vi "RunStatistics.vi"() -> ()   [LabVIEW 2018]
uses:
  General Libraries/statistics/StatisticsControl.ctl
  <vilib>/Utility/miscctls.llb/LVPointDoubleTypeDef.ctl
  General Libraries/statistics/OutputSelection.ctl
  typedef/StateMachineControl.ctl
  typedef/AcquisitionFrame.ctl
  Read and Save Files/FileType.ctl
  VisionLibrariesXimea/xiLib/xiLIB_64bit/xiLIB/xiCamLib/xiCam/PRM/PRM/PRM_v2.ctl
  VisionLibrariesXimea/xiLib/xiLIB_64bit/xiLIB/xiCamLib/xiCam/PRM/ACQ_TIMING_MODE/ACQ_TIMING_MODE.ctl
  C:/XIMEA/API/x64/xiApi.NETX64.dll
  General Libraries/statistics.lvlib
  General Libraries/Photon Filtering.lvlib
  General Libraries/myFFT.lvlib
  Read and Save Files/RW_Protocols.lvlib
panel:
  out "r":dbl[][][](array[numeric])
  out "ready for stat ?":bool
  in  "N average":i32=10
  out "error out":errorcluster
  in  "output type":T1
  in  "phase multiple select":i32[](listbox)=[0, 1, 2, 3]
  in  "Tab Control":T2(tab)
  in  "subimage control":T4={"2^n : x"=10, "2^n : y"=10, "lower left box Position"={"X"=1752.0, "Y"=1167.0}, "Height"=100, "Width"=100} {"2^n : y" min=1 max=13; "2^n : x" min=1 max=13}
  out "time for acquire":dbl[unit]
  out "Intensity Graph 2":u16[][](graph)
  out "FFT":dbl[][](graph)
  out "filtered  FFT":dbl[][](graph)
  in  "save stats":bool
  in  "image stat":T5
  out "Intensity Graph":dbl[][](graph)
  out "total frames":i32
  in  "Hologram array":dbl[](array[numeric])=[0.0, 0.25, 0.5, 0.75]
  out "fft cluster":T6
  in  "Run statistics":bool
  in  "Stop Button":bool
  # "edit this array to define how the hologram is implmented. For example, H = I1 - I3 + i I2 - i I3 will be define by the default value"
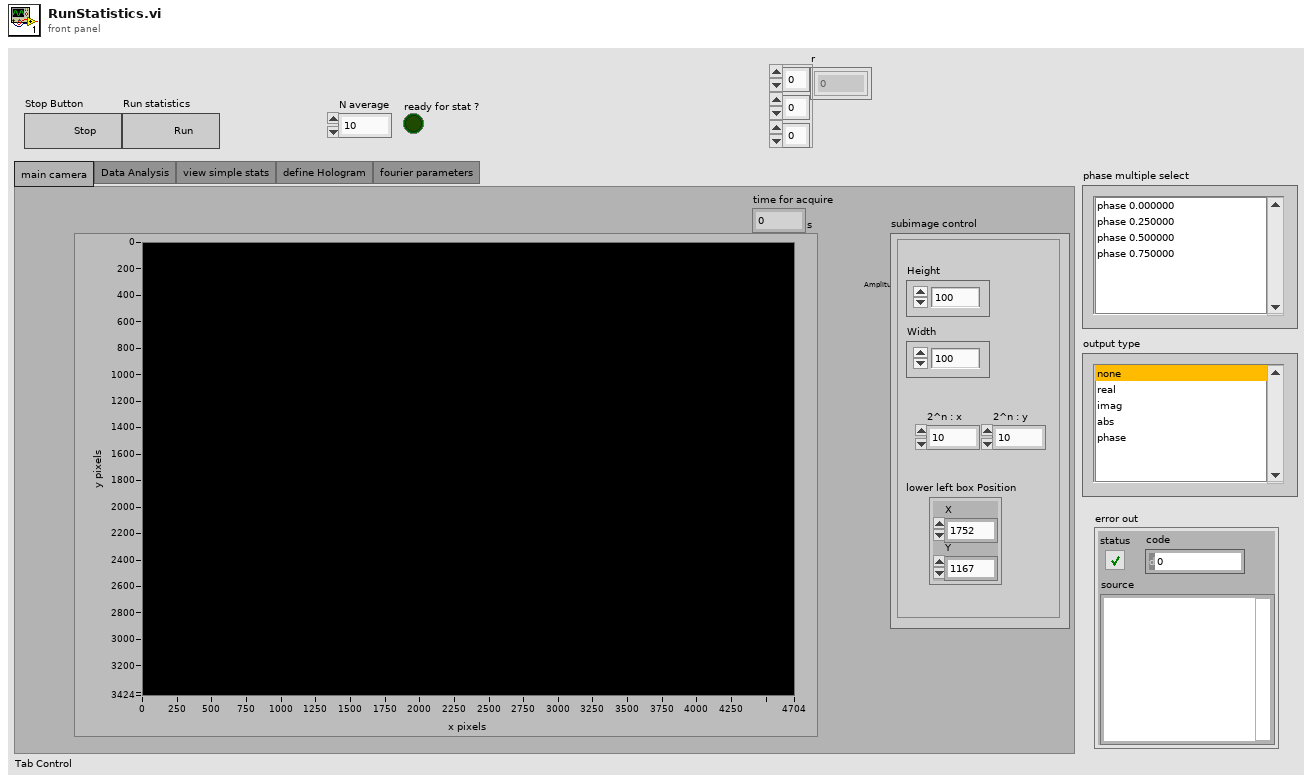
[diagram p1: front panel]
types:
  T1 = typedef "statistics.lvlib/OutputSelection.ctl" = i32
  T2 = enum32{"main camera", "Data Analysis", "view simple stats", "define Hologram", "fourier parameters"}
  T3 = typedef "LVPointDoubleTypeDef.ctl" = cluster{"X":dbl, "Y":dbl}
  T4 = cluster{"2^n : x":i8, "2^n : y":i8, "lower left box Position":T3, "Height":i32, "Width":i32}
  T5 = typedef "statistics.lvlib/StatisticsControl.ctl" = enum16{"var", "image", "SNR", "std", "average"}
  T6 = cluster{"dFx":dbl, "dFy":dbl, "Nx":i32, "Ny":i32, "FxMax":dbl, "FyMax":dbl, "Xwidth":dbl, "Ywidth":dbl, "dx":dbl, "dy":dbl, "Fx points":dbl[], "X points":dbl[], "Y points":dbl[], "Fy points":dbl[]}
  T7 = typedef "AcquisitionFrame.ctl" = cluster{"data array":u8[], "nframe":i32, "sframe":i32, "nframe0":i32, "data format":i32, "is sequence running ?":bool, "timestamp":dbl}
  T8 = typedef "StateMachineControl.ctl" = enum16{"stop acquire", "acquire sequence", "wait", "start acquire sequence", "start acquire", "acquire"}
  T9 = typedef "PRM_v2.ctl" = enum16{"ACQ_BUFFER_SIZE", "ACQ_FRAME_BURST_COUNT", "ACQ_TIMING_MODE", "ACQ_TRANSPORT_BUFFER_SIZE", "AE_MAX_LIMIT", "AEAG", "AEAG_LEVEL", "API_VERSION", "AG_MAX_LIMIT", "APPLY_CMS", "AUTO_BANDWIDTH_CALCULATION", "AUTO_WB", "AVAILABLE_BANDWIDTH", "AVAILABLE_BANDWIDTH_MAX", "AVAILABLE_BANDWIDTH_MIN", "BPC", "BUFFER_POLICY", "BUFFERS_QUEUE_SIZE", "CC_MATRIX_00", "CC_MATRIX_01", "CC_MATRIX_02", "CC_MATRIX_03", "CC_MATRIX_10", "CC_MATRIX_11", "CC_MATRIX_12", "CC_MATRIX_13", "CC_MATRIX_20", "CC_MATRIX_21", "CC_MATRIX_22", "CC_MATRIX_23", "CC_MATRIX_30", "CC_MATRIX_31", "CC_MATRIX_32", "CC_MATRIX_33", "CHIP_TEMP", "CMS", "COLOR_FILTER_ARRAY", "COOLING", "DEBOUNCE_EN", "DEBOUNCE_POL", "DEBOUNCE_T0", "DEBOUNCE_T1", "DEBUG_LEVEL", "DEFAULT_CC_MATRIX", "DEVICE_INSTANCE_PATH", "DEVICE_MODEL_ID", "DEVICE_NAME", "DEVICE_SN", "DEVICE_TYPE", "DEVICE_USER_ID", "DOWNSAMPLING", "DOWNSAMPLING_MAX", "DOWNSAMPLING_MIN", "DOWNSAMPLING_TYPE", "DRV_VERSION", "EXP_PRIORITY", "EXPOSURE", "EXPOSURE_DIRECT_UPDATE", "EXPOSURE_MAX", "EXPOSURE_MIN", "FFS_FILE_NAME", "FPGA1_VERSION", "FRAMERATE", "FRAMERATE_MAX", "FRAMERATE_MIN", "FREE_FFS_SIZE", "GAIN", "GAIN_DIRECT_UPDATE", "GAIN_MAX", "GAIN_MIN", "GAMMAC", "GAMMAY", "GPI_LEVEL", "GPI_MODE", "GPI_SELECTOR", "GPI_SELECTOR_MAX", "GPI_SELECTOR_MIN", "GPO_MODE", "GPO_SELECTOR", "GPO_SELECTOR_MAX", "GPO_SELECTOR_MIN", "HDR", "HDR_T1", "HDR_T2", "HEIGHT", "HEIGHT_MAX", "HEIGHT_MIN", "HOUSE_TEMP", "IMAGE_DATA_FORMAT", "IMAGE_IS_COLOR", "INPUT_CMS_PROFILE", "IS_COOLED", "IS_DEVICE_EXIST", "KNEEPOINT1", "KNEEPOINT2", "LED_MODE", "LED_SELECTOR", "LED_SELECTOR_MAX", "LED_SELECTOR_MIN", "LIMIT_BANDWIDTH", "LIMIT_BANDWIDTH_MAX", "LIMIT_BANDWIDTH_MIN", "LUT_EN", "LUT_INDEX", "LUT_INDEX_MAX", "LUT_INDEX_MIN", "LUT_VALUE", "LUT_VALUE_MAX", "LUT_VALUE_MIN", "MANUAL_WB", "MCU1_VERSION", "MCU2_VERSION", "OFFSET_X", "OFFSET_X_MAX", "OFFSET_X_MIN", "OFFSET_Y", "OFFSET_Y_MAX", "OFFSET_Y_MIN", "OUTPUT_CMS_PROFILE", "OUTPUT_DATA_BIT_DEPTH", "OUTPUT_DATA_PACKING", "READ_FILE_FFS", "RECENT_FRAME", "SENSOR_DATA_BIT_DEPTH", "SENSOR_MODE", "SENSOR_TAPS", "SHARPNESS", "SHUTTER_TYPE", "TARGET_TEMP", "TRG_DELAY", "TRG_SELECTOR", "TRG_SOFTWARE", "TRG_SOURCE", "USED_FFS_SIZE", "WB_KB", "WB_KG", "WB_KR", "WIDTH", "WIDTH_MAX", "WIDTH_MIN", "WRITE_FILE_FFS", "ACQ_BUFFER_SIZE_UNIT", "ACQ_TRANSPORT_BUFFER_COMMIT", "AEAG_ROI_HEIGHT", "AEAG_ROI_OFFSET_X", "AEAG_ROU_OFFSET_Y", "AEAG_ROI_WIDTH", "API_CONTEXT_LIST", "BINNING_HORIZONTAL", "BINNING_SELECTOR", "BINNING_VERTICAL", "COLUMN_FPN_CORRECTION", "COUNTER_SELECTOR", "COUNTER_VALUE", "DECIMATION_HORIZONTAL", "DECIMATION_SELECTOR", "DECIMATION_VERTICAL", "DEVICE_ID", "DEVICE_LOCATION_PATH", "DEVICE_MANIFEST", "DEVICE_RESET", "DEVICE_SENS_SN", "EXPOSURE_BURST_COUNT", "FFS_ACCESS_KEY", "GAIN_SELECTOR", "HW_REVISION", "IMAGE_BLACK_LEVEL", "IMAGE_DATA_BIT_DEPTH", "IMAGE_DATA_FORMAT_RGB32_ALPHA", "IMAGE_PAYLOAD_SIZE", "LENS_APERTURE_VALUE", "LENS_FEATURE", "LENS_FEATURE_SELECTOR", "LENS_FOCAL_LENGTH", "LENS_FOCUS_DISTANCE", "LENS_FOCUS_MOVE", "LENS_FOCUS_MOVEMENT_VALUE", "LENS_MODE", "OUTPUT_DATA_PACKING_TYPE", "SENSOR_CLOCK_FREQ_HZ", "SENSOR_CLOCK_FREQ_INDEX", "SENSOR_FEATURE_SELECTOR", "SENSOR_FEATURE_VALUE", "SENSOR_OUTPUT_CHANNEL_COUNT", "TRANSPORT_PIXEL_FORMAT", "TS_RST_MODE", "TS_RST_SOURCE"}
  T10 = typedef "ACQ_TIMING_MODE.ctl" = enum16{"FREE_RUN", "FRAME_RATE"}
  T11 = typedef "RW_Protocols.lvlib/FileType.ctl" = enum16{"png", "csv", "tiff", "dat", "bin", "txt"}
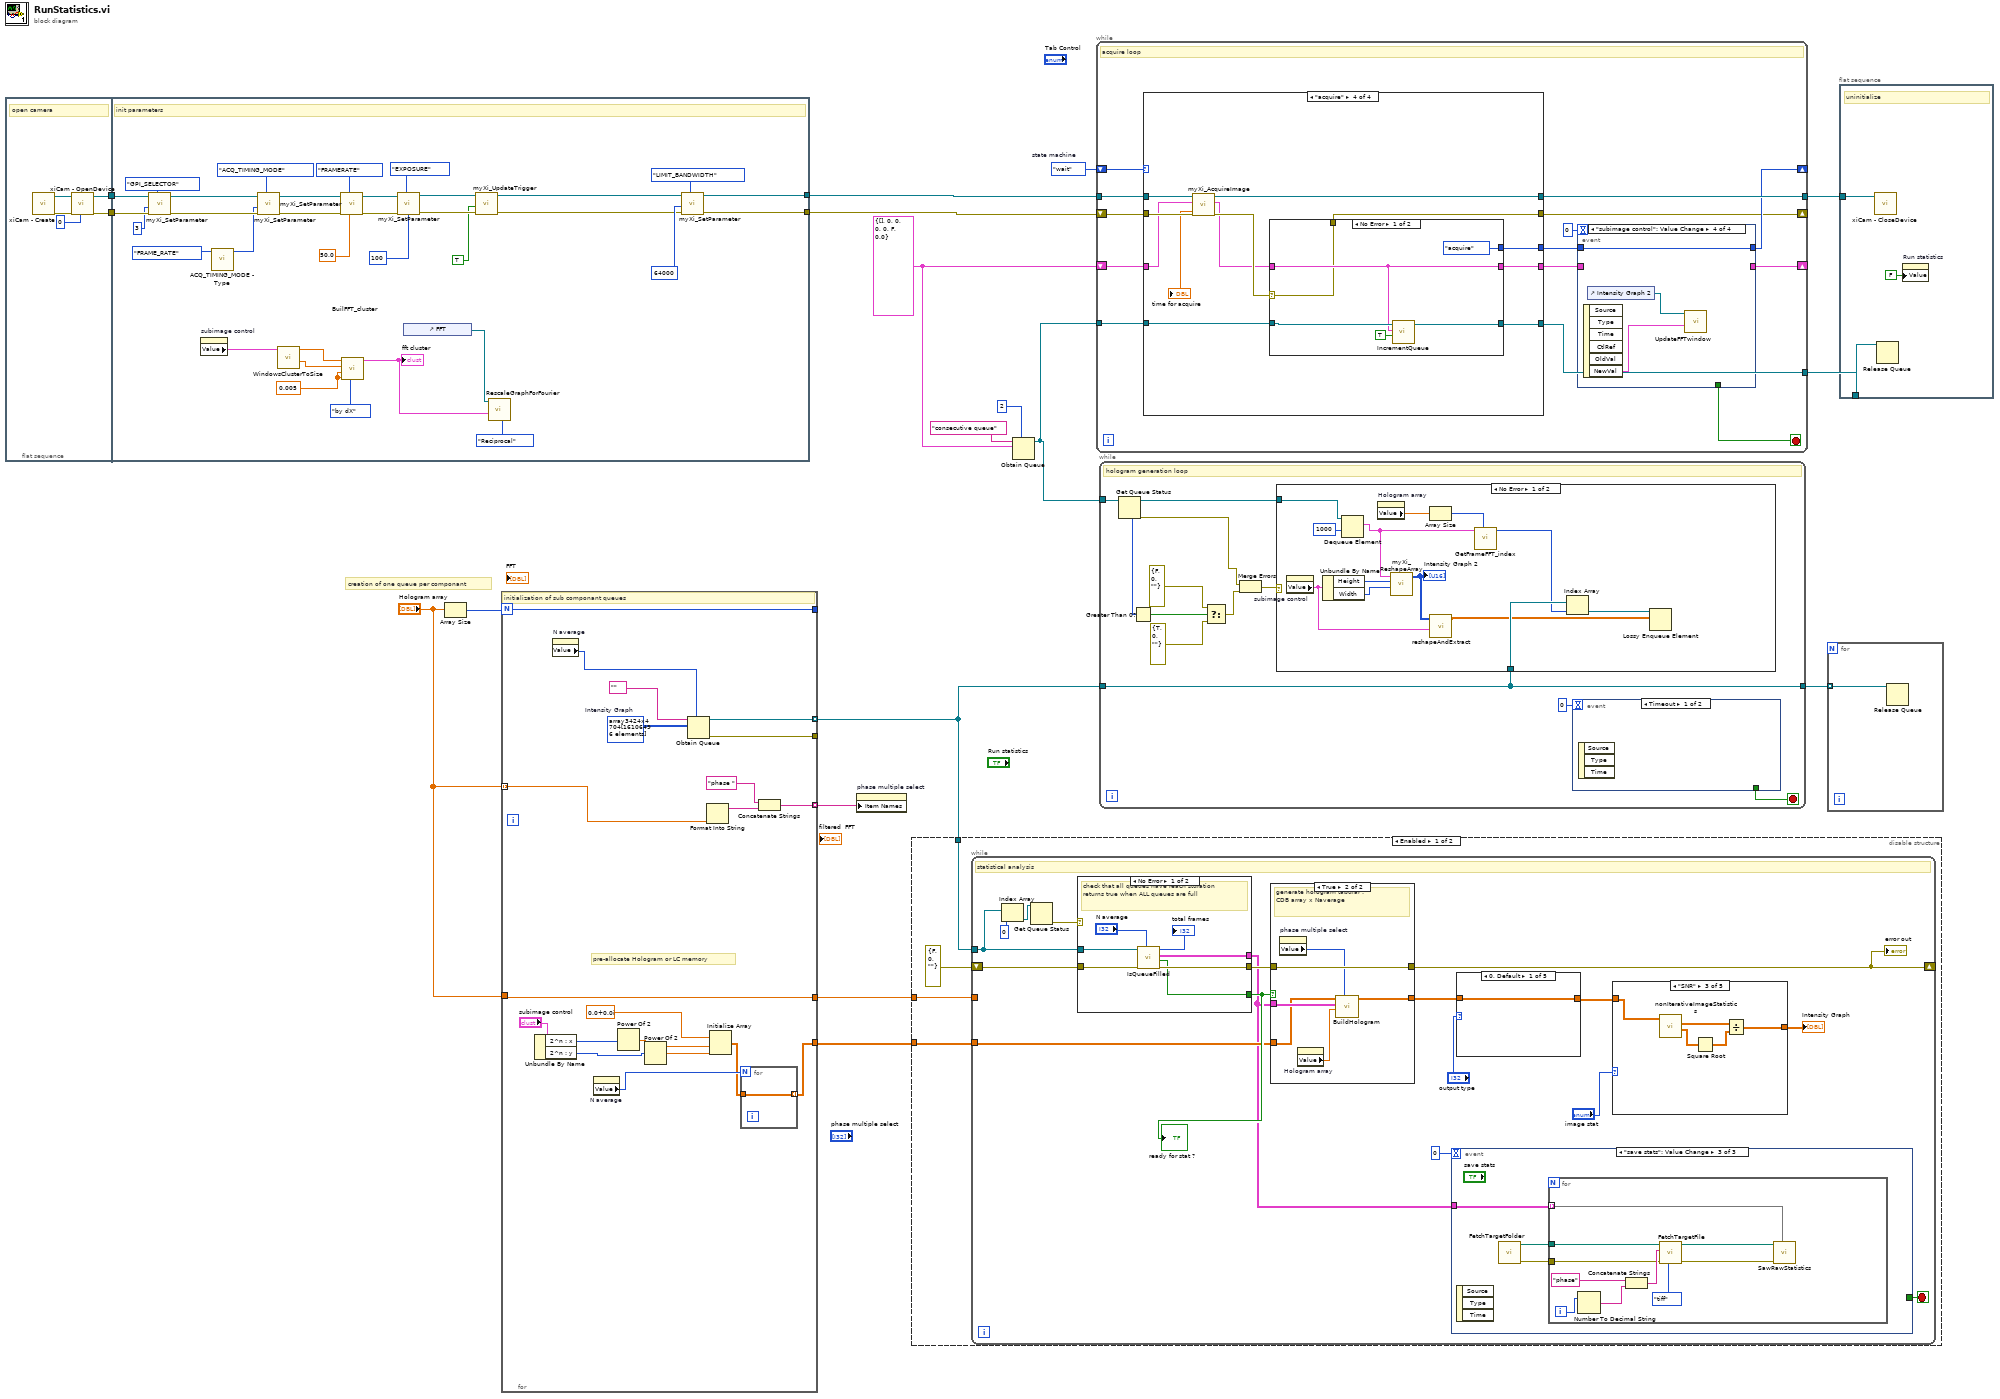
[diagram p0: block diagram]
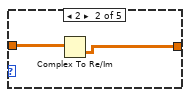
[diagram p2: hidden frame]
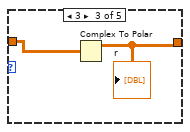
[diagram p3: hidden frame]
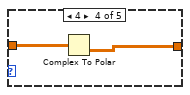
[diagram p4: hidden frame]
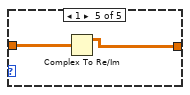
[diagram p5: hidden frame]
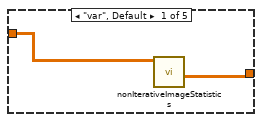
[diagram p6: hidden frame]
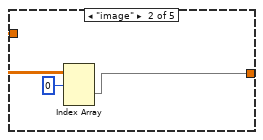
[diagram p7: hidden frame]
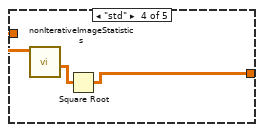
[diagram p8: hidden frame]
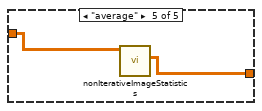
[diagram p9: hidden frame]
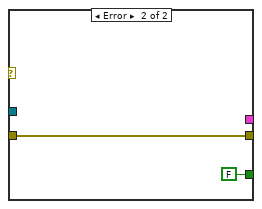
[diagram p11: hidden frame]
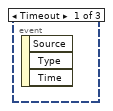
[diagram p12: hidden frame]
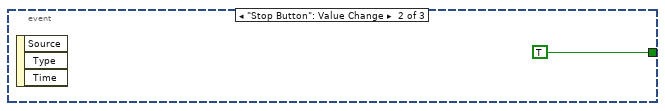
[diagram p13: hidden frame]
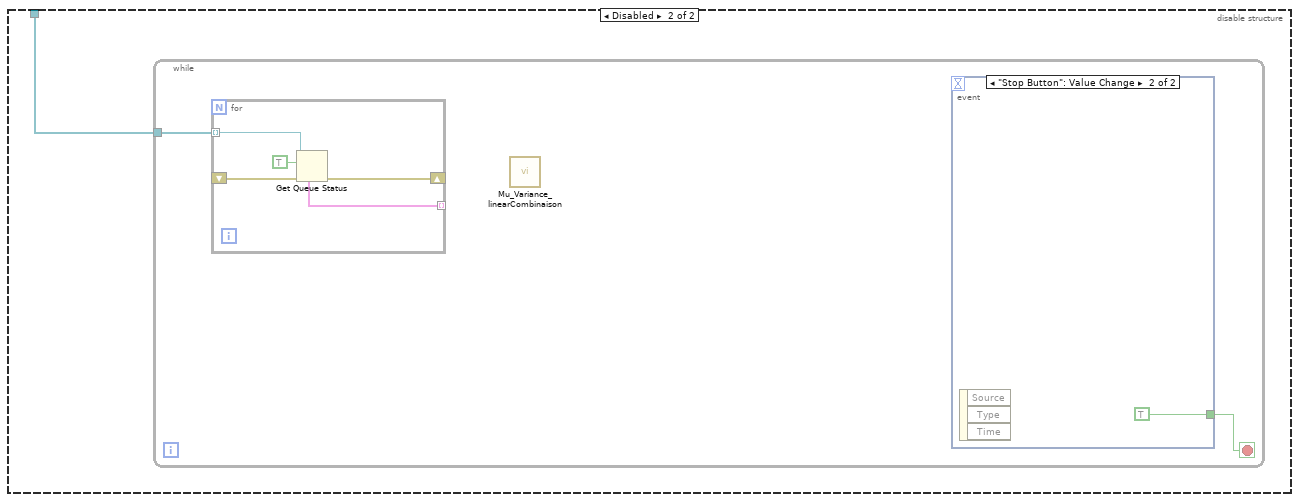
[diagram p14: hidden frame]
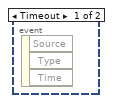
[diagram p15: hidden frame]
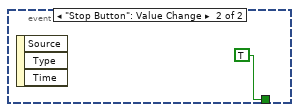
[diagram p17: hidden frame]
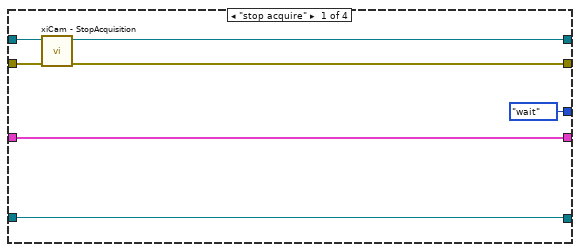
[diagram p18: hidden frame]
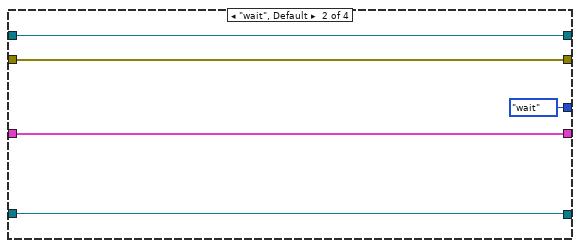
[diagram p19: hidden frame]
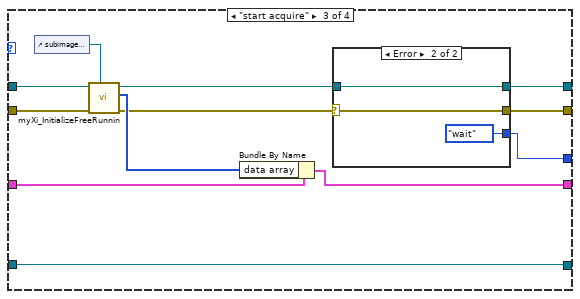
[diagram p20: hidden frame]
diagram:
  w1 = T7 {"data array"=[], "nframe"=0, "sframe"=0, "nframe0"=0, "data format"=0, "is sequence running ?"=FALSE, "timestamp"=0.0} ("acquisition frame")
  w13 = StateMachineControl."wait"  # state machine
  # "creation of one queue per componant"
  n1 = flat-sequence {
    tunnel: [w20] -> w18
    tunnel: [w19] -> w17
    tunnel: w18 -> [w56]
    tunnel: w17 -> [w57]
    tunnel: [w33] -> w16
    tunnel: [w34] -> w15
    frame #0 {
      # "open camera"
      n2 = call "xiCam - Create.vi"() -> ("error out"=w22:errorcluster, "new xiCam"=w23:refnum<k24>)  [unwired: 10 in]
      n3 = call "xiCam - OpenDevice.vi"("DevID"=0, "error in (no error)"=w22, "xiCam In"=w23) -> ("error out"=w19:errorcluster, "xiCam Out"=w20:refnum<k24>)  [unwired: 7 in]
    }
    frame #1 {
      w31 = 0.005 ("input X")
      # "init parameters"
      n4 = call "myXi_SetParameter.vi"("input PRM"=PRM_v2."GPI_SELECTOR", "error in"=w57, "input value I32"=i64 3, "xiCam IN"=w56) -> ("error out"=w53:errorcluster, "xiCam Out"=w52:refnum<k24>)  [unwired: 6 in]
      n5 = property on="subimage control" class="Clust (strict)"() -> ("Value"=w25:T4)  [unwired: 2 in, 2 out]
      n6 = call "ACQ_TIMING_MODE - Type.vi"("ACQ TIMING MODE"=ACQ_TIMING_MODE."FRAME_RATE") -> ("ACQ_TIMING_MODE_VALUE"=w50:i32)  [unwired: 9 in, 1 out]
      n7 = call "myXi_SetParameter.vi"("input PRM"=PRM_v2."ACQ_TIMING_MODE", "error in"=w53, "input value I32"=w50, "xiCam IN"=w52) -> ("error out"=w43:errorcluster, "xiCam Out"=w44:refnum<k24>)  [unwired: 6 in]
      n8 = call "WindowsClusterToSize.vi"("subwindow control 2"=w25) -> ("Ny"=w30:dbl, "Nx"=w29:dbl)  [unwired: 9 in]
      n9 = call "myXi_SetParameter.vi"("input value DBL"=sgl 50.0, "input PRM"=PRM_v2."FRAMERATE", "error in"=w43, "xiCam IN"=w44) -> ("error out"=w41:errorcluster, "xiCam Out"=w42:refnum<k24>)  [unwired: 6 in]
      n10 = call "BuilFFT_cluster.vi"("Enum"=enum16{"by dF", "by dX"}."by dX", "input Y"=w31, "input X"=w31, "Ny"=w30, "Nx"=w29) -> ("fft cluster"=w27:T6)  [unwired: 6 in]
      "fft cluster" <- w27
      n11 = call "myXi_SetParameter.vi"("input PRM"=PRM_v2."EXPOSURE", "error in"=w41, "input value I32"=i64 100, "xiCam IN"=w42) -> ("error out"=w39:errorcluster, "xiCam Out"=w40:refnum<k24>)  [unwired: 6 in]
      n12 = control-ref of="FFT"() -> (w24:refnum<vi>)
      n13 = call "myXi_UpdateTrigger.vi"("error in (no error)"=w39, "trigger"=TRUE, "xiCam IN"=w40) -> ("error out"=w35:errorcluster, "xiCam Out"=w32:refnum<k24>)  [unwired: 7 in]
      n14 = call "RescaleGraphForFourier.vi"("fft reference"=w24, "fft cluster"=w27, "Enum"=enum16{"Reciprocal", "Real"}."Reciprocal") -> ()  [unwired: 8 in]
      n15 = call "myXi_SetParameter.vi"("input PRM"=PRM_v2."LIMIT_BANDWIDTH", "error in"=w35, "input value I32"=i64 64000, "xiCam IN"=w32) -> ("error out"=w34:errorcluster, "xiCam Out"=w33:refnum<k24>)  [unwired: 6 in]
    }
  }
  n16 = Array Size(array="Hologram array") -> (size(s)=w8:i32)
  n17 = for {
    N: w8 -> [w70]
    tunnel: [w77] -> w6 mode=indexing
    tunnel: [w75] -> _
    tunnel: [w73] -> w5 mode=indexing
    tunnel: [w70] -> _
    tunnel: "Hologram array" -> [w69]
    tunnel: [w69] -> w4
    tunnel: "Hologram array" -> [w68] mode=indexing
    tunnel: [w63] -> w2
    w74 = u16[][] array3424x4704[16106496 elements]  # Intensity Graph
    # "pre-allocate Hologram or LC memory"
    # "initialization of sub componant queues"
    n18 = Unbundle By Name("subimage control") -> ("2^n : x"=w62:i8, "2^n : y"=w60:i8)
    n19 = property on="N average" class="DigNum (strict)"() -> ("Value"=w58:i32)  [unwired: 2 in, 2 out]
    n20 = property on="N average" class="DigNum (strict)"() -> ("Value"=w65:i32)  [unwired: 2 in, 2 out]
    n21 = Power Of 2(x=w62) -> (2^x=w61:dbl)
    n22 = Power Of 2(x=w60) -> (2^x=w59:dbl)
    n23 = Obtain Queue(max queue size (-1, unlimited)=w58, name (unnamed)="", element data type=w74) -> (queue out=w77:refnum<queue>, error out=w75:errorcluster)  [unwired: 2 in, 1 out]
    n24 = Format Into String(w68) -> (resulting string=w72:string)  [unwired: 3 in, 1 out]
    n25 = Initialize Array(cdb 0.0+0.0i, w61, w59) -> (w64:cdb[][])
    n26 = for {
      N: w65 -> [_]
      tunnel: w64 -> [w78]
      tunnel: [w78] -> w63 mode=indexing
    }
    n27 = Concatenate Strings("phase ", w72) -> (w73:string)
  }
  n28 = property on="phase multiple select" class="LstBox (strict)"("Item Names"=w5) -> ()  [unwired: 2 in, 2 out]
  n29 = disable-structure shown="Enabled" {
    disable-tunnel: w6 -> [w82 w155]
    disable-tunnel: w4 -> [w81 _]
    disable-tunnel: w2 -> [w79 _]
    frame Enabled {
      n30 = while {
        tunnel: w82 -> [w96]
        shift-right: [w90] -> _
        shift-left: errorcluster {"status"=FALSE, "code"=0, "source"=""} ("error out") -> [w97]
        tunnel: w81 -> [_]
        tunnel: w79 -> [w89]
        stop <- w98 stop-if-true
        # "statistical analysis"
        n31 = Index Array(array=w96, index=0) -> (element=w94:refnum<queue>)
        n32 = Get Queue Status(queue=w94) -> (error out=w93:errorcluster)  [unwired: 2 in, 7 out]
        n33 = case shown="No Error" w93 {
          tunnel: w97 -> [w138 w140]
          tunnel: [w137 w140] -> w91
          tunnel: w96 -> [w132 _]
          tunnel: [w135 FALSE ("ready for stat ?")] -> w92
          tunnel: [w134 _] -> w83
          frame No Error {
            # "check that all queues have reach sturation\nreturns true when ALL queues are full"
            n34 = call "IsQueueFilled.vi"("N average"="N average", "error in (no error)"=w138, "Array 2"=w132) -> ("error out"=w137:errorcluster, "ready for stat ?"=w135:bool, "elements"=w134:cluster{"Intensity Graph 3":u8[][]}[][], "sum"=→"total frames":i32)  [unwired: 5 in]
          }
          frame Error {
          }
        }
        "ready for stat ?" <- w92
        n35 = case shown="True" w92 {
          tunnel: w91 -> [w125 w131]
          tunnel: [w125 w131] -> w90
          tunnel: w89 -> [w124 w127]
          tunnel: [w124 w129] -> w84
          tunnel: w83 -> [_ w128]
          frame False {
          }
          frame True {
            # "generate hologram tabular :\nCDB array x Naverage"
            n36 = property on="phase multiple select" class="LstBox (strict)"() -> ("Value"=w130:i32[])  [unwired: 2 in, 2 out]
            n37 = property on="Hologram array" class="Arr (strict)"() -> ("Value"=w126:dbl[])  [unwired: 2 in, 2 out]
            n38 = call "BuildHologram.vi"("phase multiple select"=w130, "Hologram array"=w126, "elements"=w128, "pre-allocated HOL"=w127) -> ("HOL out"=w129:cdb[][][])  [unwired: 7 in]
          }
        }
        "error out" <- w90
        n39 = event shown="[2] \"save stats\": Value Change" {
          selector: _ -> [_ _ _]
          dyn-events: _ -> [_ _ _]
          timeout: 0 -> [_ _ _]
          tunnel: [_ TRUE _] -> w98
          tunnel: w83 -> [_ _ w144]
          event Timeout {
            n40 = event-data() -> ()  [unwired: 1 in, 3 out]
          }
          event "Stop Button": Value Change {
            n41 = event-data() -> ()  [unwired: 1 in, 3 out]
          }
          event "save stats": Value Change {
            n42 = event-data() -> ()  [unwired: 1 in, 3 out]
            n43 = call "FetchTargetFolder.vi"() -> ("error out"=w142:errorcluster, "Full File Path"=w143:path)  [unwired: 10 in]
            n44 = for {
              tunnel: w144 -> [w146] mode=indexing
              tunnel: w143 -> [w149]
              tunnel: w142 -> [w150]
              i -> [w154]
              n45 = Number To Decimal String(number=w154) -> (decimal integer string=w152:string)  [unwired: 1 in]
              n46 = Concatenate Strings("phase", w152) -> (w151:string)
              n47 = call "FetchTargetFile.vi"("file type"=FileType."tiff", "error in (no error)"=w150, "FileName"=w151, "Target Folder"=w149) -> ("error out"=w147:errorcluster, "Full File Path"=w148:path)  [unwired: 6 in]
              n48 = call "SawRawStatistics.vi"("elements 2"=w146, "error in (no error)"=w147, "Full File Path"=w148) -> ()  [unwired: 8 in, 1 out]
            }
          }
        }
        n49 = case shown="0, Default" "output type" {
          tunnel: w84 -> [w100 w102 w104 w106 w107]
          tunnel: [w100 w101 w103 w105 w108] -> w85
          frame 0, Default {
          }
          frame 2 {
            n50 = Complex To Re/Im(x + iy=w102) -> (y=w101:dbl[][][])  [unwired: 1 out]
          }
          frame 3 {
            n51 = Complex To Polar(r * e^(i*theta)=w104) -> (r=w103:dbl[][][])  [unwired: 1 out]
            "r" <- w103
          }
          frame 4 {
            n52 = Complex To Polar(r * e^(i*theta)=w106) -> (theta=w105:dbl[][][])  [unwired: 1 out]
          }
          frame 1 {
            n53 = Complex To Re/Im(x + iy=w107) -> (x=w108:dbl[][][])  [unwired: 1 out]
          }
        }
        n54 = case shown="\"SNR\"" "image stat" {
          tunnel: [w109 w111 w114 w119 w122] -> w87
          tunnel: w85 -> [w110 w113 w118 w121 w123]
          frame "var", Default {
            n55 = call "nonIterativeImageStatistics.vi"("HOL in"=w110) -> ("var n+1"=w109:dbl[][])  [unwired: 9 in, 1 out]
          }
          frame "image" {
            n56 = Index Array(array=w113, index (dim 0)=0 ("index (page)")) -> (element=w111:cdb[][])  [unwired: 2 in]
          }
          frame "SNR" {
            n57 = call "nonIterativeImageStatistics.vi"("HOL in"=w118) -> ("var n+1"=w117:dbl[][], "MU n+1"=w116:dbl[][])  [unwired: 9 in]
            n58 = Square Root(x=w117) -> (sqrt(x)=w115:dbl[][])
            n59 = Divide(x=w116, y=w115) -> (x/y=w114:dbl[][])
          }
          frame "std" {
            n60 = call "nonIterativeImageStatistics.vi"("HOL in"=w121) -> ("var n+1"=w120:dbl[][])  [unwired: 9 in, 1 out]
            n61 = Square Root(x=w120) -> (sqrt(x)=w119:dbl[][])
          }
          frame "average" {
            n62 = call "nonIterativeImageStatistics.vi"("HOL in"=w123) -> ("MU n+1"=w122:dbl[][])  [unwired: 9 in, 1 out]
          }
        }
        "Intensity Graph" <- w87
      }
    }
    frame Disabled {
      n63 = while {
        tunnel: w155 -> [w156]
        stop <- w157 stop-if-true
        n64 = for {
          tunnel: w156 -> [w162] mode=indexing
          shift-right: [w159] -> _
          shift-left: _ -> [w160]
          tunnel: [w158] -> _ mode=indexing
          n65 = Get Queue Status(queue=w162, return elements? (F)=TRUE, error in (no error)=w160) -> (error out=w159:errorcluster, elements=w158:cluster{"Intensity Graph":u16[][]}[])  [unwired: 6 out]
        }
        n66 = call "Mu_Variance_linearCombinaison.vi"() -> ()  [unwired: 12 in]
        n67 = event shown="[1] \"Stop Button\": Value Change" {
          selector: _ -> [_ _]
          dyn-events: _ -> [_ _]
          timeout: _ -> [_ _]
          tunnel: [_ TRUE] -> w157
          event Timeout {
            n68 = event-data() -> ()  [unwired: 1 in, 3 out]
          }
          event "Stop Button": Value Change {
            n69 = event-data() -> ()  [unwired: 1 in, 3 out]
          }
        }
      }
    }
  }
  n70 = Obtain Queue(max queue size (-1, unlimited)=2, name (unnamed)="consecutive queue", element data type=w1) -> (queue out=w10:refnum<queue>)  [unwired: 2 in, 2 out]
  n71 = while {
    tunnel: w16 -> [w173]
    tunnel: [w172] -> w14
    shift-right: [w167] -> _
    shift-left: w13 -> [w175]
    shift-right: [w170] -> _
    shift-left: w1 -> [w171]
    shift-right: [w164] -> _
    shift-left: w15 -> [w174]
    tunnel: w10 -> [w166]
    tunnel: [w165] -> w11
    stop <- w177 stop-if-true
    # "acquire loop"
    n72 = case shown="\"acquire\"" w175 {
      tunnel: w174 -> [w182 w187 w201 w220]
      tunnel: w173 -> [w183 w186 w199 w221]
      tunnel: [w181 w186 w198 w219] -> w172
      tunnel: w171 -> [w184 w189 w197 w218]
      tunnel: [w184 w189 w196 w214] -> w169
      tunnel: [StateMachineControl."wait" ("state machine") StateMachineControl."wait" ("state machine") w195 w216] -> w168
      tunnel: [w180 w187 w194 w210] -> w164
      tunnel: w166 -> [w178 w185 w193 w213]
      tunnel: [w178 w185 w193 w212] -> w165
      frame "stop acquire" {
        n73 = call "xiCam - StopAcquisition.vi"("error in (no error)"=w182, "xiCam In"=w183) -> ("error out"=w180:errorcluster, "xiCam Out"=w181:refnum<k24>)  [unwired: 8 in]
      }
      frame "wait", Default {
      }
      frame "start acquire" {
        n74 = control-ref of="subimage control"() -> (w192:refnum<vi>)
        n75 = call "myXi_InitializeFreeRunnin.vi"("subimage IN"=w192, "error in (no error)"=w201, "xiCam IN"=w199) -> ("error out"=w190:errorcluster, "Array"=w191:u8[], "xiCam Out"=w200:refnum<k24>)  [unwired: 6 in]
        n76 = Bundle By Name(cluster=w197, "data array"=w191) -> (w196:T7)
        n77 = case shown="Error" w190 {
          selector: w190 -> [w203 w208]
          tunnel: w200 -> [w206 w209]
          tunnel: [w205 w209] -> w198
          tunnel: [w204 StateMachineControl."wait" ("state machine")] -> w195
          tunnel: [w202 w208] -> w194
          frame No Error {
            w204 = StateMachineControl."acquire"  # state machine
            n78 = invoke class="xiCam" method="StartAcquisition"(reference=w206, error in=w203) -> (reference out=w205:refnum<k24>, error out=w202:errorcluster)  [unwired: 1 in, 1 out]
          }
          frame Error {
          }
        }
      }
      frame "acquire" {
        n79 = call "myXi_AcquireImage.vi"("error in"=w220, "acquisition frame"=w218, "xiCam In"=w221) -> ("error out"=w217:errorcluster, "acquisition frame out"=w215:T7, "xiCam Out"=w219:refnum<k24>, "time for acquire"=→"time for acquire":dbl[unit])  [unwired: 4 in, 1 out]
        n80 = case shown="No Error" w217 {
          selector: w217 -> [w222 w229]
          tunnel: [StateMachineControl."acquire" ("state machine") w230] -> w216
          tunnel: w215 -> [w224 w233]
          tunnel: [w224 w233] -> w214
          tunnel: w213 -> [w226 w232]
          tunnel: [w223 w232] -> w212
          tunnel: [w222 w228] -> w210
          frame No Error {
            n81 = call "IncrementQueue.vi"("is sequence running ?"=TRUE, "acquisition frame"=w224, "queue in"=w226) -> ("queue out"=w223:refnum<queue>)  [unwired: 8 in]
          }
          frame Error {
            n82 = Unbundle By Name(w229) -> ("code"=w231:i32)
            n83 = case shown="1172" w231 {
              tunnel: [StateMachineControl."wait" ("state machine") StateMachineControl."acquire" ("state machine")] -> w230
              tunnel: w229 -> [w234 _]
              tunnel: [w234 errorcluster {"status"=FALSE, "code"=0, "source"=""} ("error IO")] -> w228
              frame 0, Default {
              }
              frame 1172 {
              }
            }
          }
        }
      }
    }
    n84 = event shown="[3] \"subimage control\": Value Change" {
      selector: _ -> [_ _ _ _]
      dyn-events: _ -> [_ _ _ _]
      timeout: 0 -> [_ _ _ _]
      tunnel: [_ TRUE _ _] -> w177
      tunnel: [w238 w240 w244 _] -> w170
      tunnel: w169 -> [w238 w240 w244 _]
      tunnel: w168 -> [w239 _ _ w250]
      tunnel: [w239 StateMachineControl."wait" ("state machine") w243 w250] -> w167
      event Timeout {
        n85 = event-data() -> ()  [unwired: 1 in, 3 out]
      }
      event "Stop Button": Value Change {
        n86 = event-data() -> ()  [unwired: 1 in, 6 out]
      }
      event "Run statistics": Value Change {
        n87 = event-data() -> ("NewVal"=w245:bool)  [unwired: 1 in, 5 out]
        n88 = case shown="True" w245 {
          tunnel: [w246 StateMachineControl."start acquire" ("state machine")] -> w243
          frame False {
            w246 = StateMachineControl."stop acquire"  # state machine
          }
          frame True {
          }
        }
      }
      event "subimage control": Value Change {
        n89 = event-data() -> ("NewVal"=w249:T4)  [unwired: 1 in, 5 out]
        n90 = control-ref of="Intensity Graph 2"() -> (w248:refnum<vi>)
        n91 = call "UpdateFFTwindow.vi"("subwindow IN"=w249, "Intensity Graph"=w248) -> ()  [unwired: 9 in, 1 out]
      }
    }
  }
  n92 = while {
    tunnel: w10 -> [w257]
    tunnel: w6 -> [w253]
    tunnel: [w253] -> w7
    stop <- w261 stop-if-true
    # "hologram generation loop"
    n93 = Get Queue Status(queue=w257) -> (queue out=w254:refnum<queue>, error out=w252:errorcluster, # elements in queue=w255:i32)  [unwired: 2 in, 5 out]
    n94 = Greater Than 0?(x=w255) -> (x > 0?=w260:bool)
    n95 = Select(t=errorcluster {"status"=FALSE, "code"=0, "source"=""} ("error constant"), s=w260, f=errorcluster {"status"=TRUE, "code"=0, "source"=""} ("error constant")) -> (s? t:f=w251:errorcluster)
    n96 = Merge Errors(w252, w251) -> (w256:errorcluster)
    n97 = case shown="No Error" w256 {
      tunnel: w254 -> [w275 _]
      tunnel: w253 -> [w273 _]
      frame No Error {
        n98 = property on="subimage control" class="Clust (strict)"() -> ("Value"=w263:T4)  [unwired: 2 in, 2 out]
        n99 = Unbundle By Name(w263) -> ("Height"=w267:i32, "Width"=w266:i32)
        n100 = Dequeue Element(queue=w275, timeout in ms (-1)=1000) -> (element=w268:T7)  [unwired: 1 in, 3 out]
        n101 = property on="Hologram array" class="Arr (strict)"() -> ("Value"=w272:dbl[])  [unwired: 2 in, 2 out]
        n102 = call "myXi_ReshapeArray.vi"("width"=w266, "height"=w267, "acquisition frame"=w268) -> ("output array"=w264:u16[][])  [unwired: 8 in]
        "Intensity Graph 2" <- w264
        n103 = Array Size(array=w272) -> (size(s)=w271:i32)
        n104 = call "reshapeAndExtract.vi"("window"=w263, "output array"=w264) -> ("subarray"=w265:dbl[][])  [unwired: 9 in]
        n105 = call "GetFrameFFT_index.vi"("sframe Max"=w271, "element"=w268) -> ("index out"=w270:i32)  [unwired: 8 in, 1 out]
        n106 = Index Array(array=w273, index=w270) -> (element=w269:refnum<queue>)
        n107 = Lossy Enqueue Element(queue=w269, element=w265) -> ()  [unwired: 1 in, 4 out]
      }
      frame Error {
      }
    }
    n108 = event shown="[0] Timeout" {
      selector: _ -> [_ _]
      dyn-events: _ -> [_ _]
      timeout: 0 -> [_ _]
      tunnel: [_ TRUE] -> w261
      event Timeout {
        n109 = event-data() -> ()  [unwired: 1 in, 3 out]
      }
      event "Stop Button": Value Change {
        n110 = event-data() -> ()  [unwired: 1 in, 3 out]
      }
    }
  }
  n111 = for {
    tunnel: w7 -> [w277] mode=indexing
    n112 = Release Queue(queue=w277) -> ()  [unwired: 2 in, 3 out]
  }
  n113 = flat-sequence {
    tunnel: w14 -> [w280]
    tunnel: w11 -> [w279]
    frame #0 {
      # "uninitialize"
      n114 = call "xiCam - CloseDevice.vi"("xiCam In"=w280) -> ()  [unwired: 10 in, 1 out]
      n115 = Release Queue(queue=w279) -> ()  [unwired: 2 in, 3 out]
      n116 = property on="Run statistics" class="Bool (strict)"("Value"=FALSE ("Run statistics")) -> ()  [unwired: 2 in, 2 out]
    }
  }
